vi "cmd_build.vi"(7 "command":T1, 8 "error  in":errorcluster, 11 "payload":u8[](array[numeric]) format="0x%x") -> (0 "out":errorcluster, 3 "cmd":string)   [LabVIEW 2019]
uses:
  type_cmd.ctl
panel:
  out "checksumm":u8 format="0x%x"
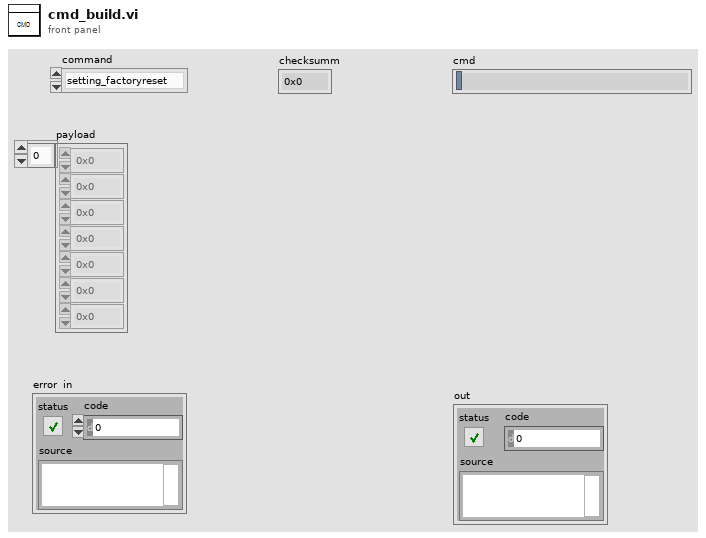
[diagram p1: front panel]
types:
  T1 = typedef "type_cmd.ctl" = enum16{"setting_factoryreset", "setting_justworks", "scan_getdevices", "scan_stop", "scan_start", "send", "disconnect", "connect"}
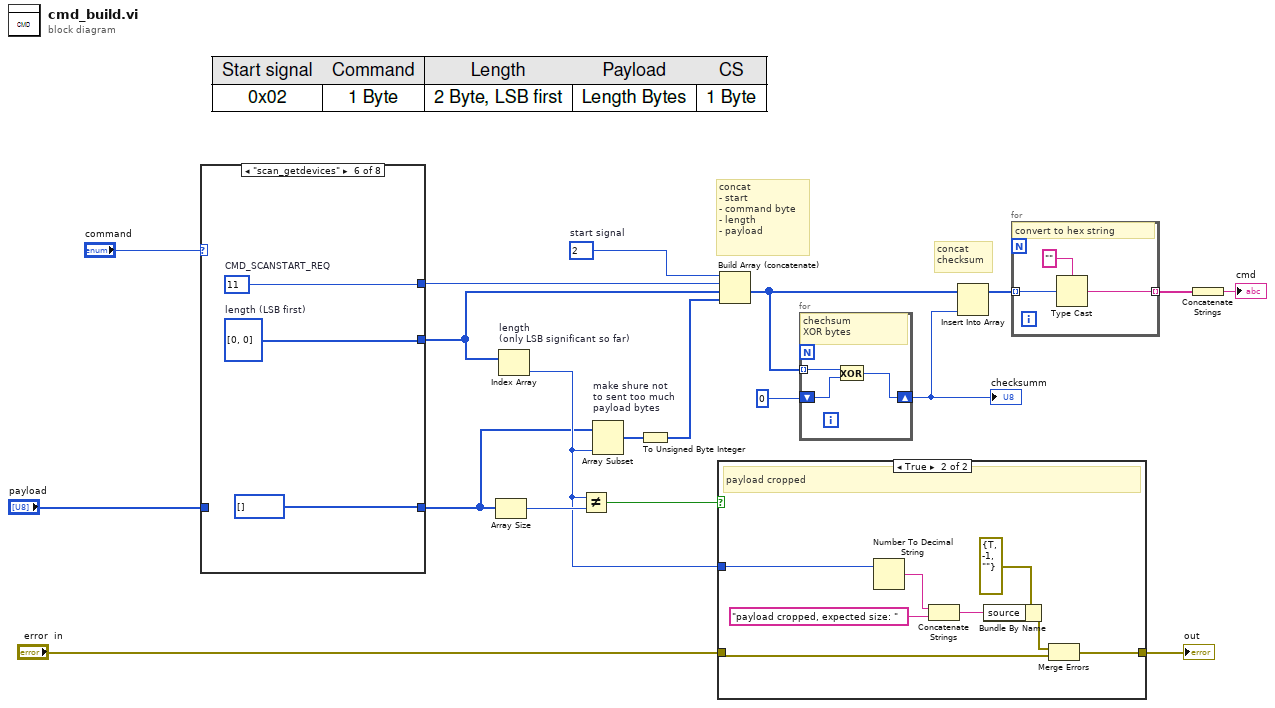
[diagram p0: block diagram]
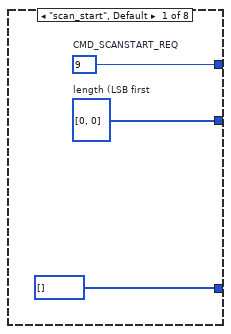
[diagram p3: hidden frame]
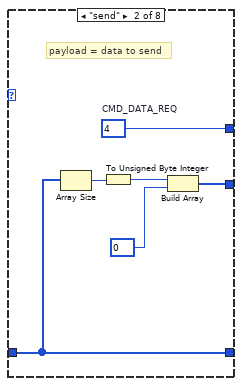
[diagram p4: hidden frame]
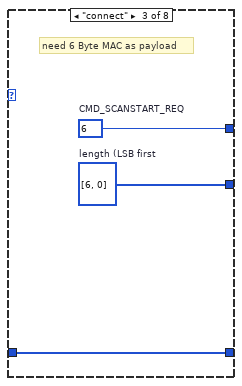
[diagram p5: hidden frame]
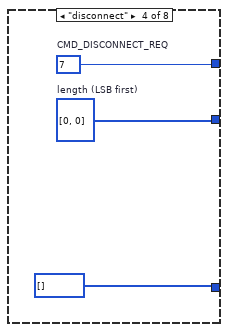
[diagram p6: hidden frame]
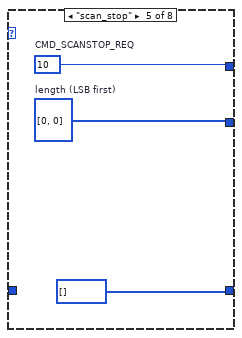
[diagram p7: hidden frame]
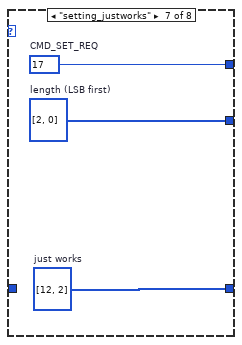
[diagram p8: hidden frame]
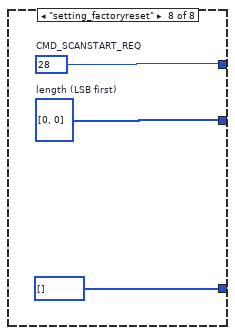
[diagram p9: hidden frame]
diagram:
  w19 = u8 2  # start signal
  # "concat \nchecksum"
  # "concat \n- start \n- command byte\n- length\n- payload"
  n1 = case shown="\"scan_getdevices\"" "command" {
    tunnel: [w22 w28 w31 w34 w37 w40 w43 w46] -> w18
    tunnel: [w21 w26 w30 w33 w36 w39 w42 w45] -> w17
    tunnel: "payload" -> [_ w23 w29 _ _ _ _ _]
    tunnel: [u8[] [] ("just works") w23 w29 u8[] [] ("just works") u8[] [] ("just works") u8[] [] ("just works") w41 u8[] [] ("just works")] -> w1
    frame "scan_start", Default {
      w21 = u8[] [0, 0]  # length (LSB first
      w22 = u8 9  # CMD_SCANSTART_REQ
    }
    frame "send" {
      w28 = u8 4  # CMD_DATA_REQ
      # "payload = data to send"
      n2 = Array Size(array=w23) -> (size(s)=w25:i32)
      n3 = To Unsigned Byte Integer(number=w25) -> (unsigned 8bit integer=w24:u8)
      n4 = Build Array(w24, u8 0) -> (w26:u8[])
    }
    frame "connect" {
      w30 = u8[] [6, 0]  # length (LSB first
      w31 = u8 6  # CMD_SCANSTART_REQ
      # "need 6 Byte MAC as payload"
    }
    frame "disconnect" {
      w33 = u8[] [0, 0]  # length (LSB first)
      w34 = u8 7  # CMD_DISCONNECT_REQ
    }
    frame "scan_stop" {
      w36 = u8[] [0, 0]  # length (LSB first)
      w37 = u8 10  # CMD_SCANSTOP_REQ
    }
    frame "scan_getdevices" {
      w39 = u8[] [0, 0]  # length (LSB first)
      w40 = u8 11  # CMD_SCANSTART_REQ
    }
    frame "setting_justworks" {
      w41 = u8[] [12, 2]  # just works
      w42 = u8[] [2, 0]  # length (LSB first)
      w43 = u8 17  # CMD_SET_REQ
    }
    frame "setting_factoryreset" {
      w45 = u8[] [0, 0]  # length (LSB first)
      w46 = u8 28  # CMD_SCANSTART_REQ
    }
  }
  n5 = Array Size(array=w1) -> (size(s)=w16:i32)
  n6 = Index Array "length\n(only LSB significant so far)"(array=w17) -> (element=w3:u8)  [unwired: 1 in]
  n7 = Not Equal?(x=w3, y=w16) -> (x != y?=w10:bool)
  n8 = Array Subset "make shure not \nto sent too much \npayload bytes"(array=w1, length=w3) -> (w12:u8[])  [unwired: 1 in]
  n9 = To Unsigned Byte Integer(number=w12) -> (unsigned 8bit integer=w11:u8[])
  n10 = case shown="True" w10 {
    tunnel: "error  in" -> [w47 w55]
    tunnel: [w47 w54] -> w8
    tunnel: w3 -> [_ w53]
    frame False {
    }
    frame True {
      # "payload cropped"
      n11 = Number To Decimal String(number=w53) -> (decimal integer string=w50:string)  [unwired: 1 in]
      n12 = Concatenate Strings(w50, "payload cropped, expected size: " ("source")) -> (w49:string)
      n13 = Bundle By Name(cluster=errorcluster {"status"=TRUE, "code"=-1, "source"=""} ("error constant"), "source"=w49) -> (w48:errorcluster)
      n14 = Merge Errors(w48, w55) -> (w54:errorcluster)
    }
  }
  "out" <- w8
  n15 = Build Array (concatenate)(w19, w18, w17, w11) -> (w14:u8[])
  n16 = for {
    tunnel: w14 -> [w57] mode=indexing
    shift-right: [w58] -> w7
    shift-left: u8 0 -> [w56]
    # "chechsum\nXOR bytes"
    n17 = Exclusive Or(1:w56, 2:w57) -> (0:w58:u8)
  }
  "checksumm" <- w7
  n18 = Insert Into Array(array=w14, new element=w7) -> (w4:u8[])  [unwired: 1 in]
  n19 = for {
    tunnel: w4 -> [w60] mode=indexing
    tunnel: [w59] -> w5 mode=indexing
    # "convert to hex string"
    n20 = Type Cast(type="", x=w60) -> (*(type *) &x=w59:string)
  }
  n21 = Concatenate Strings(w5) -> (→"cmd":string)
